vi "Search 1D String Array.vi"   [LabVIEW 2016, in "SLL String.lvlib"]
uses:
  SLL String.lvlib
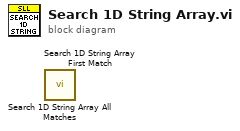
[diagram p0: block diagram]
diagram:
  n1 = call "Search 1D String Array All Matches.vi"() -> ()  [unwired: 3 in, 1 out]
  n2 = call "Search 1D String Array First Match.vi"() -> ()  [unwired: 3 in, 1 out]
